vi "LogEvents.vi"(8 "error in":errorcluster, 9 "Start time":u32, 11 "refnum in":refnum<file>) -> (0 "error out":errorcluster, 3 "refnum out":refnum<file>)   [LabVIEW 2018]
uses:
  Framework/Robot Global Data.vi
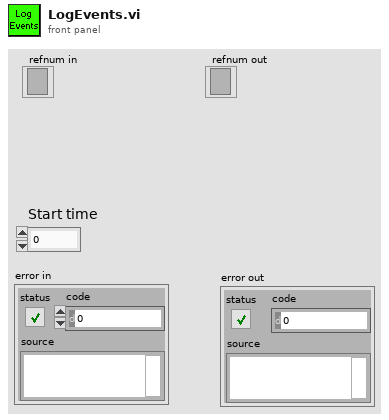
[diagram p1: front panel]
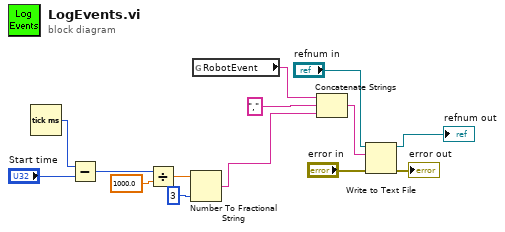
[diagram p0: block diagram]
diagram:
  n1 = Tick Count (ms)() -> (millisecond timer value=w12:u32)
  n2 = Subtract(x=w12, y="Start time") -> (x-y=w11:u32)
  n3 = Divide(x=w11, y=1000.0 ("input 9")) -> (x/y=w9:dbl)
  n4 = Number To Fractional String(number=w9, precision (6)=i16 3) -> (F-format string=w1:string)  [unwired: 2 in]
  n5 = global read "Robot Global Data.vi" "RobotEvent"() -> (w6:string)
  n6 = Concatenate Strings(w6, "," ("string"), w1) -> (w5:string)
  n7 = Write to Text File(file (use dialog)="refnum in", text=w5, error in="error in") -> (refnum out=→"refnum out":refnum<file>, error out=→"error out":errorcluster)  [unwired: 1 in, 1 out]
